vi "util_generate_actions.vi"(7 "hmi_references":T2, 8 "error in (no error)":errorcluster) -> (0 "error out":errorcluster, 3 "actions []":cluster{"index":i32, "action":T1}[](array[cluster]))   [LabVIEW 2015, in "lv-build-interface.lvlib"]
uses:
  lv-build-interface.lvlib
  _controls/hmi_references.ctl
  _controls/action.ctl
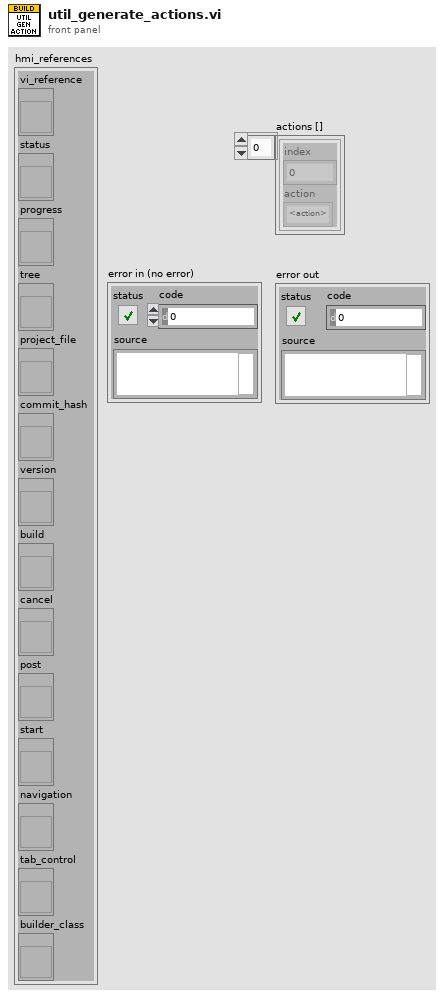
[diagram p1: front panel]
types:
  T1 = typedef "lv-build-interface.lvlib/action.ctl" = enum16{"<action>", "build", "post", "deploy", "<null>"}
  T2 = typedef "lv-build-interface.lvlib/hmi_references.ctl" = cluster{"vi_reference":refnum<vi>, "status":refnum<vi>, "progress":refnum<vi>, "tree":refnum<vi>, "project_file":refnum<vi>, "commit_hash":refnum<vi>, "version":refnum<vi>, "build":refnum<vi>, "cancel":refnum<vi>, "post":refnum<vi>, "start":refnum<vi>, "navigation":refnum<vi>, "tab_control":refnum<vi>, "builder_class":refnum<vi>}
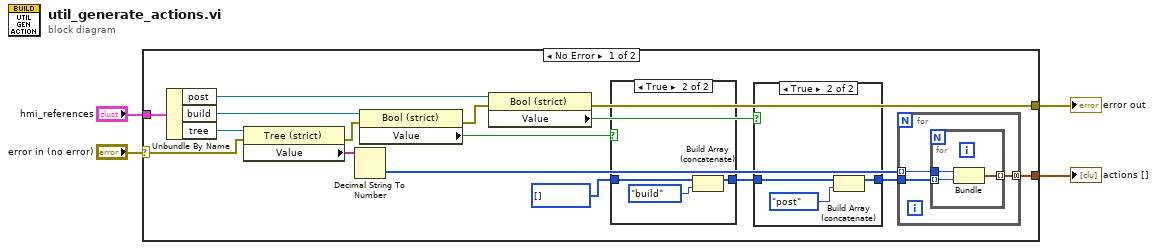
[diagram p0: block diagram]
diagram:
  n1 = case shown="No Error" "error in (no error)" {
    selector: "error in (no error)" -> [w11 w35]
    tunnel: "hmi_references" -> [w20 _]
    tunnel: [w7 _] -> w2
    tunnel: [w6 w35] -> w1
    frame No Error {
      w14 = T1[] [] items=["<action>", "build", "post", "deploy", "<null>"] ("Array")
      n2 = Unbundle By Name(w20) -> ("post"=w16:refnum<vi>, "build"=w17:refnum<vi>, "tree"=w12:refnum<vi>)
      n3 = property class="Tree (strict)"(reference=w12, error in=w11) -> (error out=w10:errorcluster, "Value"=w19:string[])  [unwired: 1 out]
      n4 = Decimal String To Number(string=w19) -> (number=w18:i32[])  [unwired: 2 in, 1 out]
      n5 = property class="Bool (strict)"(reference=w17, error in=w10) -> (error out=w15:errorcluster, "Value"=w13:bool)  [unwired: 1 out]
      n6 = property class="Bool (strict)"(reference=w16, error in=w15) -> (error out=w6:errorcluster, "Value"=w5:bool)  [unwired: 1 out]
      n7 = case shown="True" w13 {
        tunnel: w14 -> [w25 w28]
        tunnel: [w25 w27] -> w9
        frame False {
        }
        frame True {
          n8 = Build Array (concatenate)(w28, action."build" ("action")) -> (w27:T1[])
        }
      }
      n9 = case shown="True" w5 {
        tunnel: w9 -> [w21 w24]
        tunnel: [w21 w23] -> w8
        frame False {
        }
        frame True {
          n10 = Build Array (concatenate)(w24, action."post" ("action")) -> (w23:T1[])
        }
      }
      n11 = for {
        tunnel: w18 -> [w31] mode=indexing
        tunnel: [w30] -> w7 mode=concatenating
        tunnel: w8 -> [w29]
        n12 = for {
          tunnel: w31 -> [w33]
          tunnel: [w34] -> w30 mode=indexing
          tunnel: w29 -> [w32] mode=indexing
          n13 = Bundle(w33, "action"=w32) -> (w34:cluster{i32, "action":T1})  [unwired: 1 in]
        }
      }
    }
    frame Error {
    }
  }
  "error out" <- w1
  "actions []" <- w2
